vi "空调控制.vi"() -> ()   [LabVIEW 2016, in "环境动力监测库.lvlib" / "空调库.lvlib"]
uses:
  <vilib>/Utility/config.llb/NI_LVConfig.lvlib
panel:
  in  "输入簇":T1
  out "布尔 2":bool=TRUE
  in  "变更空调型号":bool
  out "布尔":bool
  # "空调监测"
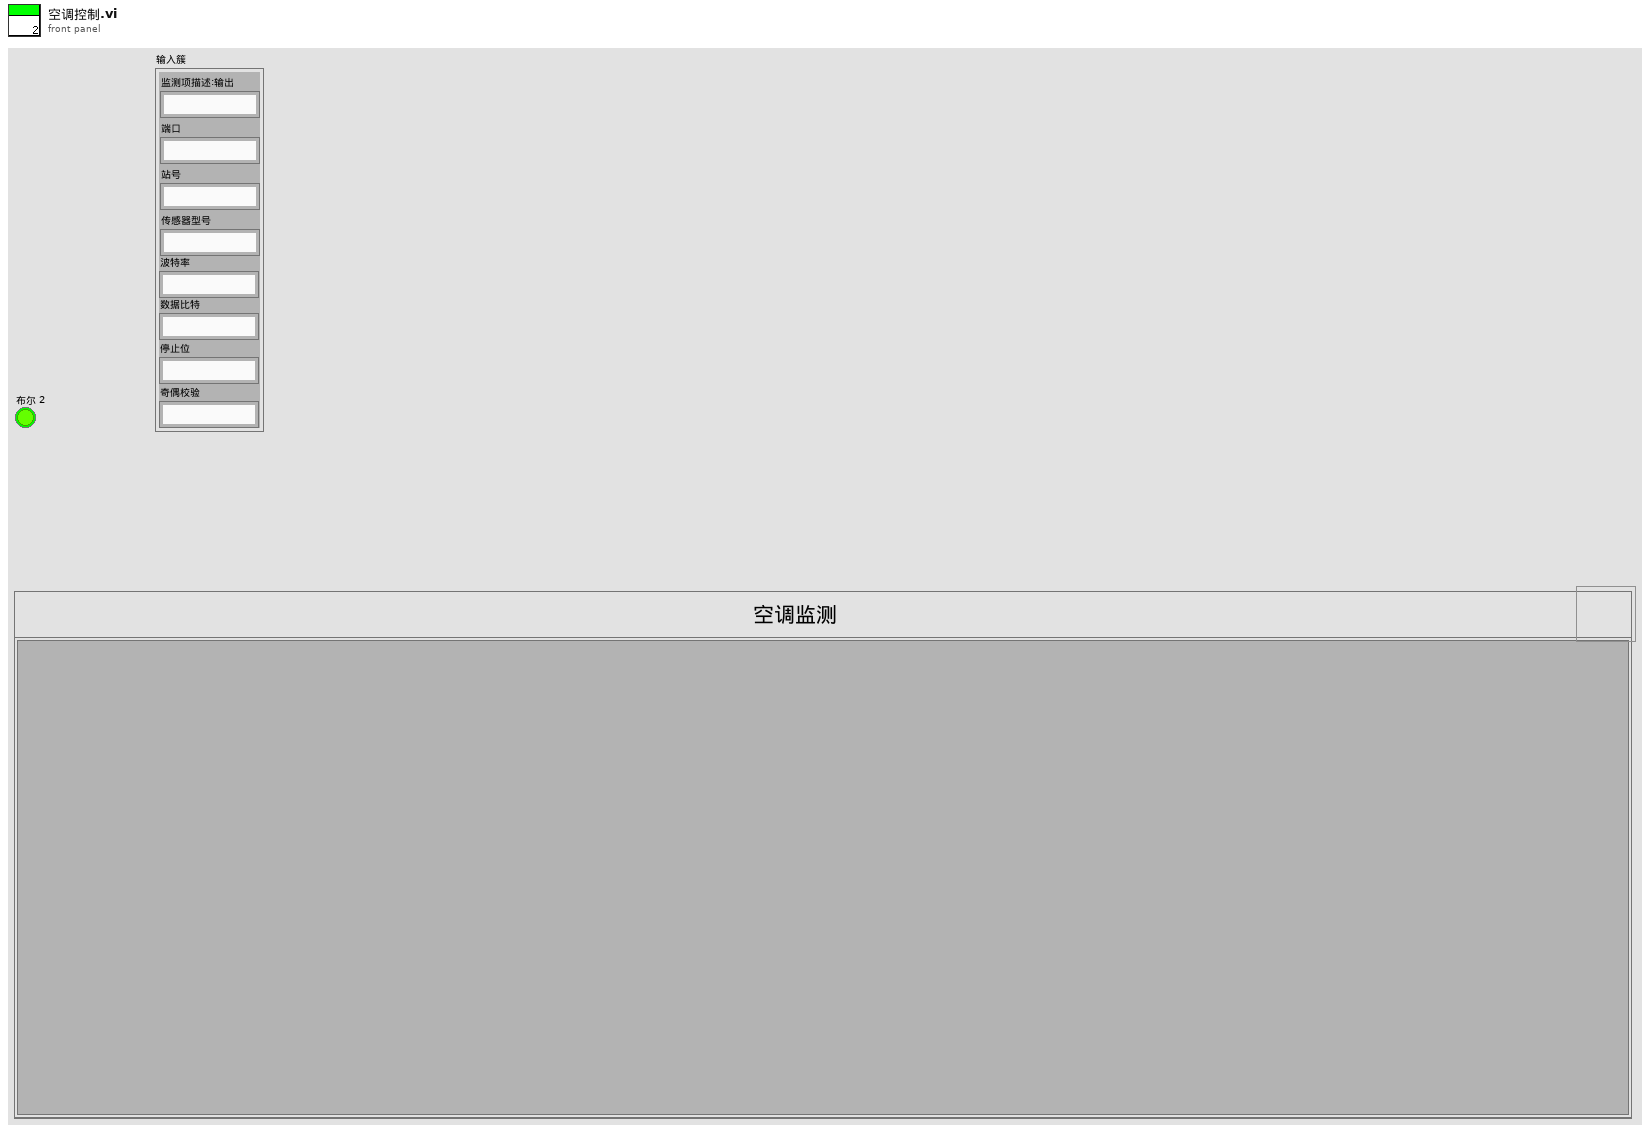
[diagram p1: front panel]
types:
  T1 = cluster{"监测项描述:输出":string, "端口":string, "站号":string, "传感器型号":string, "波特率":string, "停止位":string, "奇偶校验":string, "数据比特":string}
  T2 = cluster{"baud rate (bps)":u32, "stop bits":u16, "parity":u16, "flow control":u16, "timeout":u32, "retries":i32}
  T3 = typedef "NI_LVConfig.lvlib/Config Data RefNum.ctl" = refnum<k1>
  T4 = enum32{"Bad", "Idle", "Run top level", "Running"}
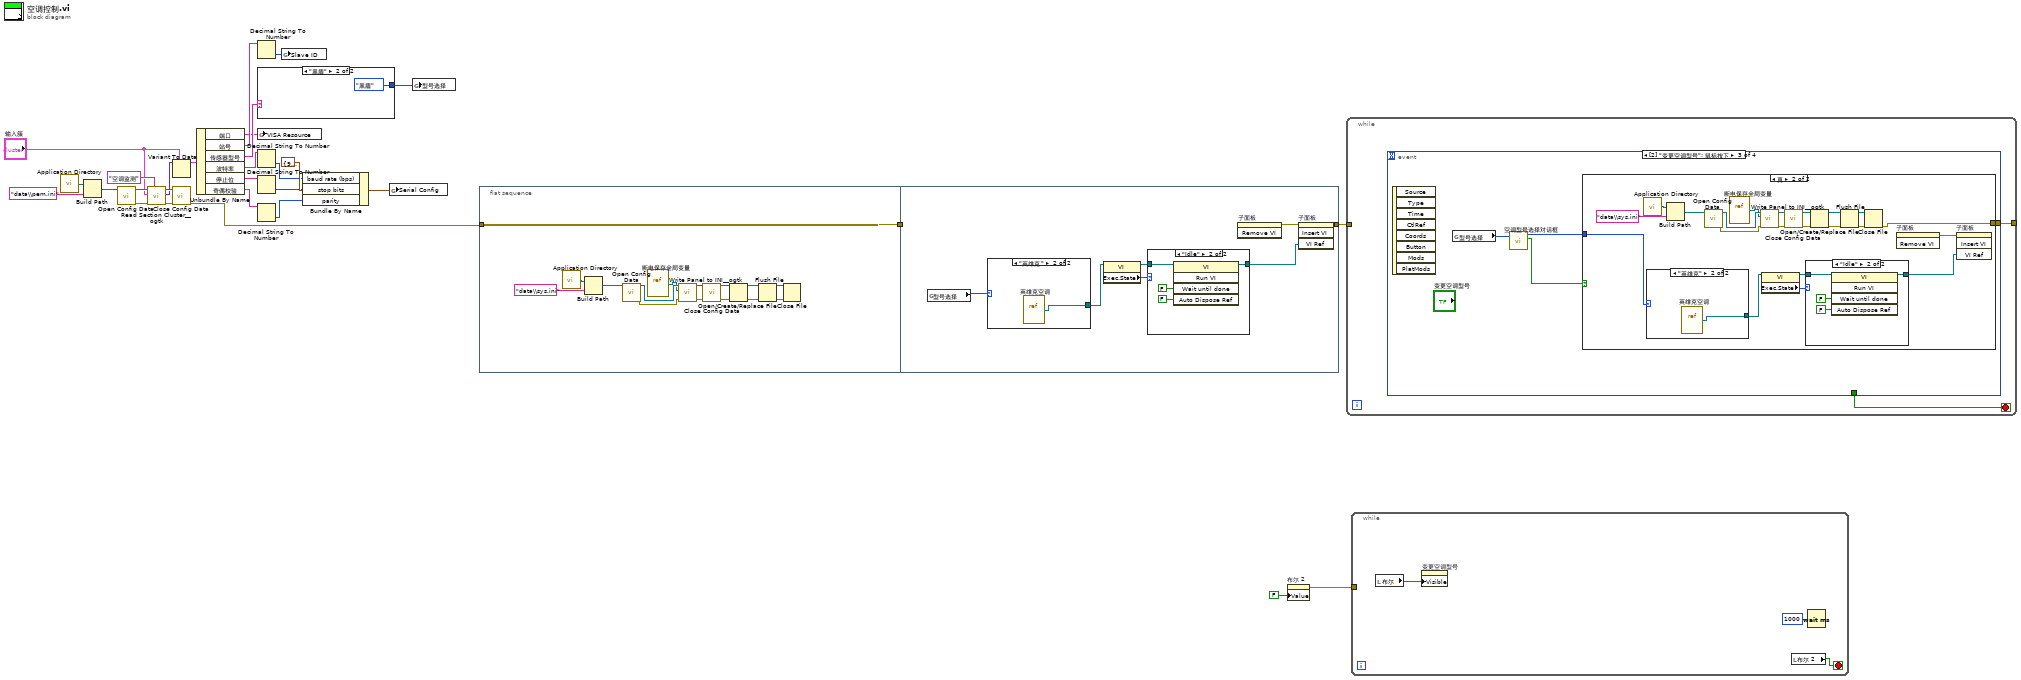
[diagram p0: block diagram]
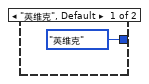
[diagram p2: hidden frame]
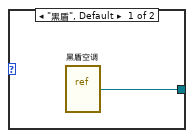
[diagram p3: hidden frame]
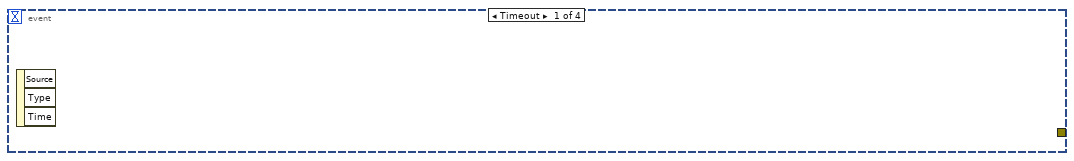
[diagram p5: hidden frame]
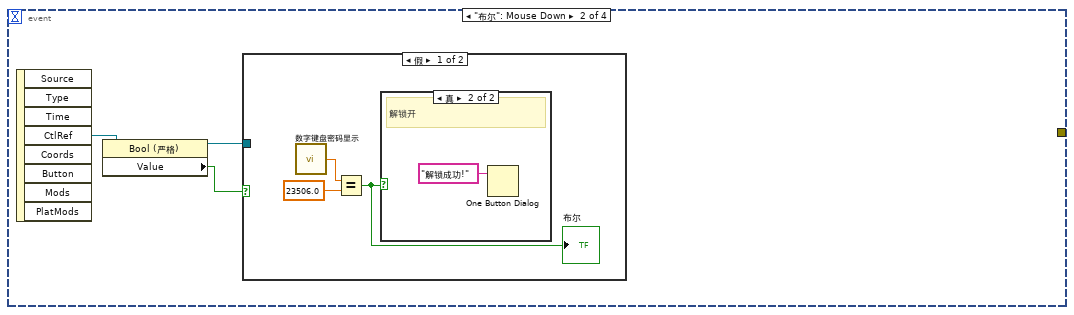
[diagram p6: hidden frame]
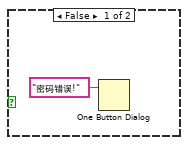
[diagram p7: hidden frame]
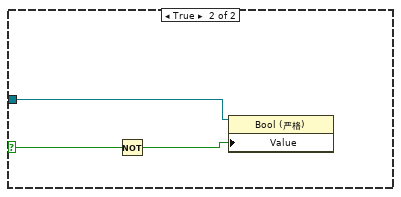
[diagram p8: hidden frame]
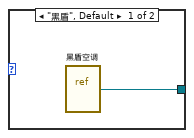
[diagram p10: hidden frame]
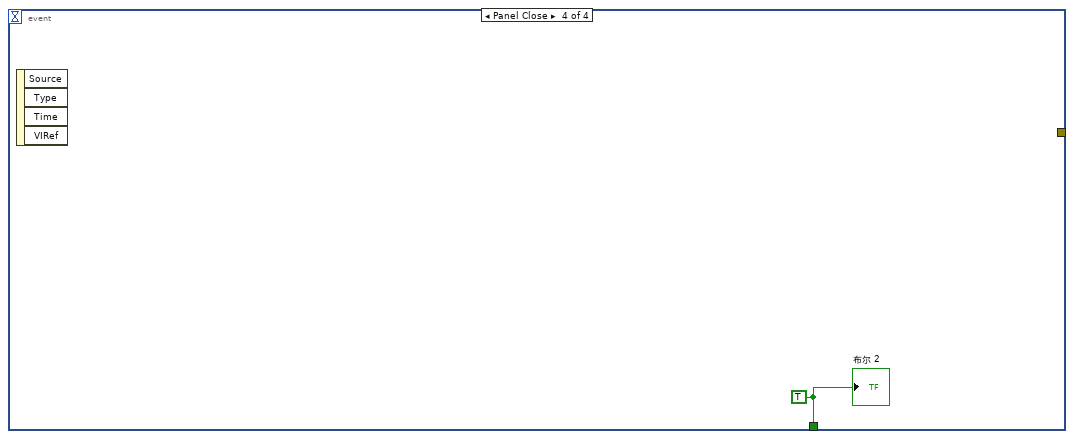
[diagram p12: hidden frame]
diagram:
  n1 = call <vilib>:"Application Directory.vi"() -> ("Application Directory"=w23:path)
  n2 = Build Path(base path=w23, name or relative path="data\\pem.ini" ("名称或相对路径")) -> (appended path=w24:path)
  n3 = call <vilib>:"Open Config Data.vi"("configuration file path"=w24) -> ("error out"=w25:errorcluster, "refnum"=w26:T3)  [unwired: 8 in, 1 out]
  n4 = call <userlib>:"Read Section Cluster__ogtk.vi"("section (optional)"="空调监测", "error in (no error)"=w25, "Section Formatted Cluster Type"="输入簇", "refnum"=w26) -> ("error out"=w19:errorcluster, "Section Formatted Cluster"=w18:variant, "dup refnum"=w20:T3)  [unwired: 3 in, 2 out]
  n5 = Variant To Data(type="输入簇", Variant=w18) -> (data=w16:T1)  [unwired: 1 in, 1 out]
  n6 = call <vilib>:"Close Config Data.vi"("error in (no error)"=w19, "refnum"=w20) -> ("error out"=w2:errorcluster)  [unwired: 8 in, 1 out]
  n7 = Unbundle By Name(w16) -> ("端口"=w11:string, "站号"=w13:string, "传感器型号"=w15:string, "波特率"=w9:string, "停止位"=w7:string, "奇偶校验"=w5:string)
  n8 = Decimal String To Number(string=w13) -> (number=w12:i32)  [unwired: 2 in, 1 out]
  n9 = case shown="\"黑盾\"" w15 {
    tunnel: [enum16{"黑盾", "英维克"}."英维克" ("型号选择") enum16{"黑盾", "英维克"}."黑盾" ("型号选择")] -> w14
    frame "英维克", Default {
    }
    frame "黑盾" {
    }
  }
  n10 = global write "断电保存全局变量.vi" "VISA Resource"(w11) -> ()
  n11 = Decimal String To Number(string=w9) -> (number=w8:i32)  [unwired: 2 in, 1 out]
  n12 = Decimal String To Number(string=w7) -> (number=w6:i32)  [unwired: 2 in, 1 out]
  n13 = Decimal String To Number(string=w5) -> (number=w4:i32)  [unwired: 2 in, 1 out]
  n14 = global write "断电保存全局变量.vi" "Slave ID"(w12) -> ()
  n15 = Bundle By Name(cluster=T2 {"baud rate (bps)"=9600, "stop bits"=10, "parity"=0, "flow control"=0, "timeout"=1000, "retries"=1} ("Serial Config"), "baud rate (bps)"=w8, "stop bits"=w6, "parity"=w4) -> (w3:T2)
  n16 = global write "断电保存全局变量.vi" "Serial Config"(w3) -> ()
  n17 = global write "断电保存全局变量.vi" "型号选择"(w14) -> ()
  n18 = flat-sequence {
    tunnel: w2 -> [w46]
    tunnel: [w46] -> w1
    tunnel: [w47] -> w29
    tunnel: w1 -> [_]
    frame #0 {
      n19 = call <vilib>:"Application Directory.vi"() -> ("Application Directory"=w44:path)
      n20 = Build Path(base path=w44, name or relative path="data\\sys.ini" ("名称或相对路径")) -> (appended path=w43:path)
      n21 = call <vilib>:"Open Config Data.vi"("configuration file path"=w43) -> ("error out"=w39:errorcluster, "refnum"=w42:T3)  [unwired: 8 in, 1 out]
      n22 = vi-ref "断电保存全局变量.vi"() -> (w41:refnum<vi>)
      n23 = call <userlib>:"Write Panel to INI__ogtk.vi"("error in (no error)"=w39, "VI ref"=w41, "refnum"=w42) -> ("error out"=w38:errorcluster, "refnum out"=w40:T3)  [unwired: 7 in]
      n24 = call <vilib>:"Close Config Data.vi"("error in (no error)"=w38, "refnum"=w40) -> ("error out"=w33:errorcluster, "file path"=w32:path)  [unwired: 8 in]
      n25 = Open/Create/Replace File(file path (use dialog)=w32, error in=w33) -> (refnum out=w36:refnum<file>, error out=w37:errorcluster)  [unwired: 4 in, 1 out]
      n26 = Flush File(refnum=w36, error in=w37) -> (refnum out=w35:refnum<file>, error out=w34:errorcluster)
      n27 = Close File(refnum=w35, error in=w34) -> ()  [unwired: 2 out]
    }
    frame #1 {
      n28 = global read "断电保存全局变量.vi" "型号选择"() -> (w49:enum16{"黑盾", "英维克"})
      n29 = case shown="\"英维克\"" w49 {
        tunnel: [w54 w55] -> w48
        frame "黑盾", Default {
          n30 = vi-ref "黑盾空调.vi"() -> (w54:refnum<vi>)
        }
        frame "英维克" {
          n31 = vi-ref "英维克空调.vi"() -> (w55:refnum<vi>)
        }
      }
      n32 = property class="VI"(reference=w48) -> (reference out=w52:refnum<vi>, "Exec.State"=w53:T4)  [unwired: 1 in, 1 out]
      n33 = case shown="\"Idle\"" w53 {
        tunnel: w52 -> [w56 w58]
        tunnel: [w56 w57] -> w50
        frame "Bad", Default {
        }
        frame "Idle" {
          n34 = invoke class="VI" method="Run VI"(reference=w58, "Wait until done"=FALSE ("结束前等待"), "Auto Dispose Ref"=FALSE ("自动销毁引用")) -> (reference out=w57:refnum<vi>)  [unwired: 2 in, 4 out]
        }
      }
      n35 = invoke on="子面板" class="SubPnl" method="Remove VI"() -> (error out=w51:errorcluster)  [unwired: 3 in, 2 out]
      n36 = invoke on="子面板" class="SubPnl" method="Insert VI"(error in=w51, "VI Ref"=w50) -> (error out=w47:errorcluster)  [unwired: 2 in, 3 out]
    }
  }
  n37 = property on="布尔 2" class="Bool (严格)"("Value"=FALSE ("布尔 2")) -> (error out=w27:errorcluster)  [unwired: 2 in, 1 out]
  n38 = while {
    tunnel: w29 -> [_]
    tunnel: [w62] -> _
    stop <- w61 stop-if-true
    n39 = event shown="[2] \"变更空调型号\": 鼠标按下" {
      selector: _ -> [_ _ _ _]
      dyn-events: _ -> [_ _ _ _]
      timeout: _ -> [_ _ _ _]
      tunnel: [_ _ w75 _] -> w62
      tunnel: [_ _ _ w106] -> w61
      event Timeout {
        n40 = event-data() -> ()  [unwired: 1 in, 3 out]
      }
      event "布尔": Mouse Down {
        n41 = event-data() -> ("CtlRef"=w65:refnum<vi>)  [unwired: 1 in, 7 out]
        n42 = property class="Bool (严格)"(reference=w65) -> (reference out=w63:refnum<vi>, "Value"=w64:bool)  [unwired: 1 in, 1 out]
        n43 = case shown="假" w64 {
          selector: w64 -> [_ w73]
          tunnel: w63 -> [_ w72]
          frame False {
            n44 = call "数字键盘密码显示.vi"() -> ("NewNumber"=w68:sgl)  [unwired: 1 in]
            n45 = Equal?(x=w68, y=sgl 23506.0) -> (x = y?=w66:bool)
            "布尔" <- w66
            n46 = case shown="真" w66 {
              frame False {
                n47 = One Button Dialog(message="密码错误!" ("消息")) -> ()  [unwired: 1 in, 1 out]
              }
              frame True {
                # "解锁开"
                n48 = One Button Dialog(message="解锁成功!" ("消息")) -> ()  [unwired: 1 in, 1 out]
              }
            }
          }
          frame True {
            n49 = Not(x=w73) -> (.not. x?=w71:bool)
            n50 = property class="Bool (严格)"(reference=w72, "Value"=w71) -> ()  [unwired: 1 in, 2 out]
          }
        }
      }
      event "变更空调型号": Mouse Down {
        n51 = event-data() -> ()  [unwired: 1 in, 8 out]
        n52 = global read "断电保存全局变量.vi" "型号选择"() -> (w74:enum16{"黑盾", "英维克"})
        n53 = call "空调型号选择对话框.vi"("枚举"=w74) -> ("布尔"=w77:bool, "枚举 2"=w76:enum16{"黑盾", "英维克"})  [unwired: 9 in]
        n54 = case shown="真" w77 {
          tunnel: w76 -> [_ w93]
          tunnel: [_ w78] -> w75
          frame False {
          }
          frame True {
            n55 = call <vilib>:"Application Directory.vi"() -> ("Application Directory"=w91:path)
            n56 = case shown="\"英维克\"" w93 {
              tunnel: [w99 w100] -> w94
              frame "黑盾", Default {
                n57 = vi-ref "黑盾空调.vi"() -> (w99:refnum<vi>)
              }
              frame "英维克" {
                n58 = vi-ref "英维克空调.vi"() -> (w100:refnum<vi>)
              }
            }
            n59 = Build Path(base path=w91, name or relative path="data\\sys.ini" ("名称或相对路径")) -> (appended path=w90:path)
            n60 = call <vilib>:"Open Config Data.vi"("configuration file path"=w90) -> ("error out"=w86:errorcluster, "refnum"=w89:T3)  [unwired: 8 in, 1 out]
            n61 = vi-ref "断电保存全局变量.vi"() -> (w88:refnum<vi>)
            n62 = call <userlib>:"Write Panel to INI__ogtk.vi"("error in (no error)"=w86, "VI ref"=w88, "refnum"=w89) -> ("error out"=w85:errorcluster, "refnum out"=w87:T3)  [unwired: 7 in]
            n63 = property class="VI"(reference=w94) -> (reference out=w97:refnum<vi>, "Exec.State"=w98:T4)  [unwired: 1 in, 1 out]
            n64 = call <vilib>:"Close Config Data.vi"("error in (no error)"=w85, "refnum"=w87) -> ("error out"=w80:errorcluster, "file path"=w79:path)  [unwired: 8 in]
            n65 = case shown="\"Idle\"" w98 {
              tunnel: w97 -> [w101 w103]
              tunnel: [w101 w102] -> w95
              frame "Bad", Default {
              }
              frame "Idle" {
                n66 = invoke class="VI" method="Run VI"(reference=w103, "Wait until done"=FALSE ("结束前等待"), "Auto Dispose Ref"=FALSE ("自动销毁引用")) -> (reference out=w102:refnum<vi>)  [unwired: 2 in, 4 out]
              }
            }
            n67 = Open/Create/Replace File(file path (use dialog)=w79, error in=w80) -> (refnum out=w83:refnum<file>, error out=w84:errorcluster)  [unwired: 4 in, 1 out]
            n68 = Flush File(refnum=w83, error in=w84) -> (refnum out=w82:refnum<file>, error out=w81:errorcluster)
            n69 = Close File(refnum=w82, error in=w81) -> (error out=w78:errorcluster)  [unwired: 1 out]
            n70 = invoke on="子面板" class="SubPnl" method="Remove VI"() -> (error out=w96:errorcluster)  [unwired: 3 in, 2 out]
            n71 = invoke on="子面板" class="SubPnl" method="Insert VI"(error in=w96, "VI Ref"=w95) -> ()  [unwired: 2 in, 4 out]
          }
        }
      }
      event Panel Close {
        w106 = TRUE
        n72 = event-data() -> ()  [unwired: 1 in, 4 out]
        "布尔 2" <- w106
      }
    }
  }
  n73 = while {
    tunnel: w27 -> [_]
    stop <- w107 stop-if-true
    n74 = local read "布尔"() -> (w108:bool)
    n75 = property on="变更空调型号" class="Bool (严格)"("Visible"=w108) -> ()  [unwired: 2 in, 2 out]
    n76 = local read "布尔 2"() -> (w107:bool)
    n77 = Wait (ms)(milliseconds to wait=u32 1000 ("等待时间（毫秒）")) -> ()  [unwired: 1 out]
  }
